vi "Read_Coil_Traces.vi"(1 "Reduction":i32=10, 2 "New Folder":path, 3 "Gas Desk Folder":path) -> ()   [LabVIEW 2010]
uses:
  Controls/Ch_and_Spans.ctl
  Globals/Meas_global.vi
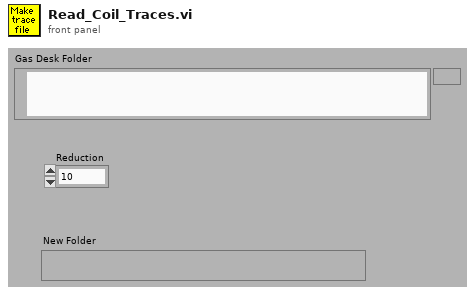
[diagram p1: front panel]
types:
  T1 = typedef "Ch_and_Spans.ctl" = cluster{"high limit (10V)":sgl, "low limit (-10V)":sgl, "Ch No":i16, "Var name":string, "Use Latest Calib":bool}
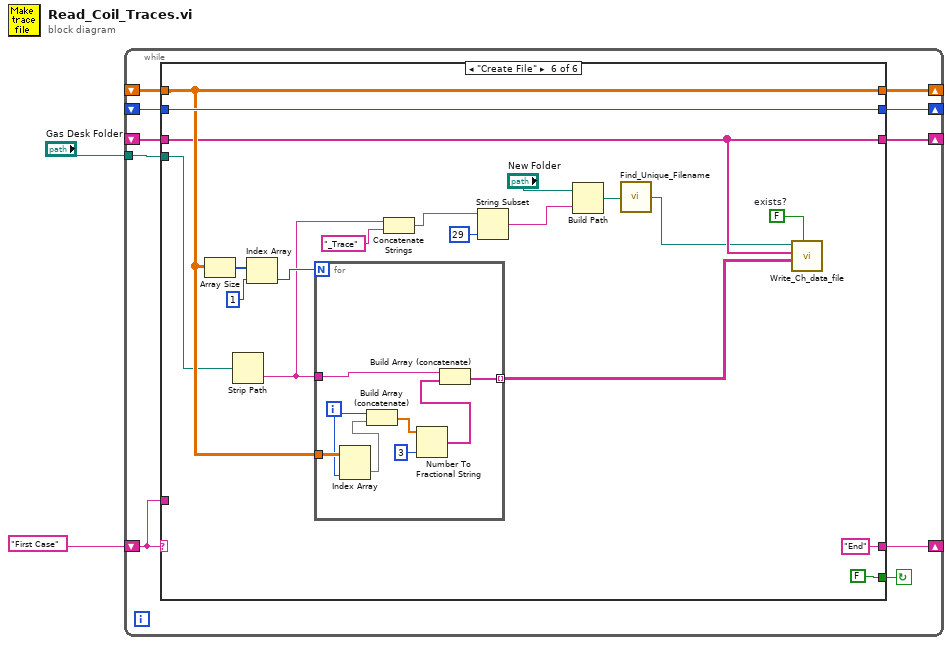
[diagram p0: block diagram]
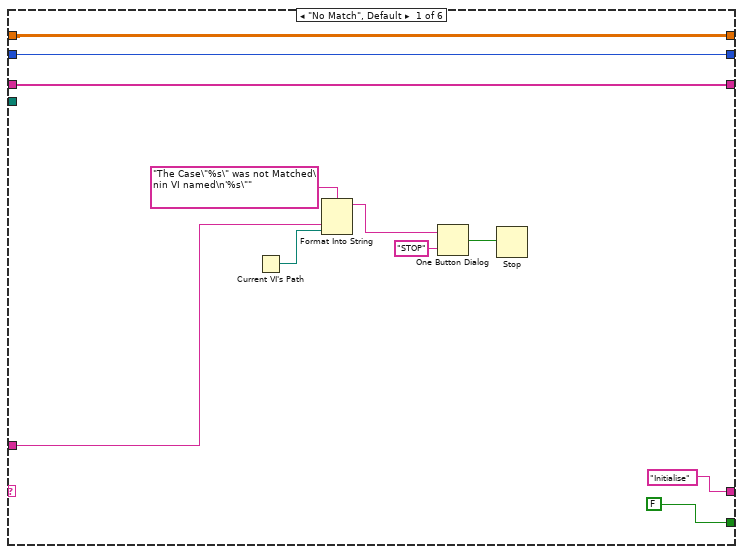
[diagram p2: hidden frame]
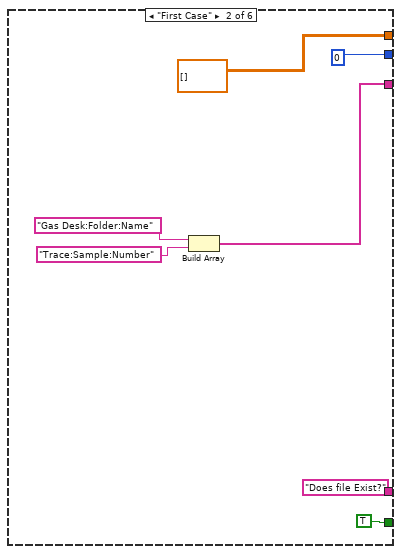
[diagram p3: hidden frame]
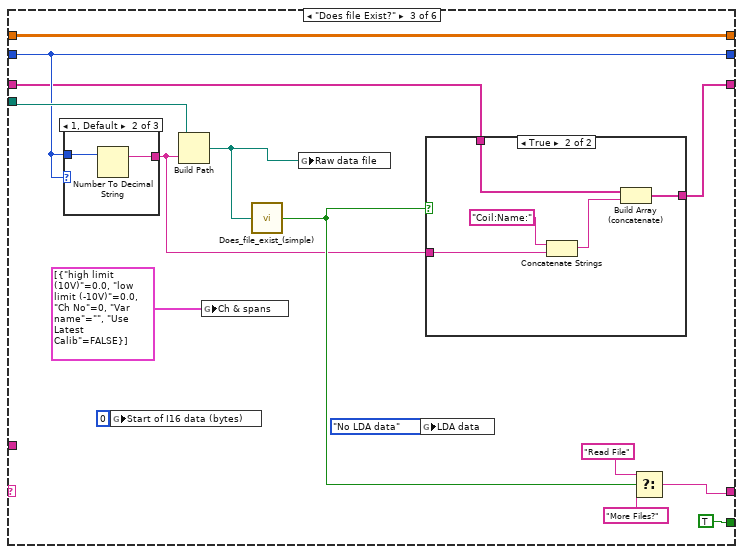
[diagram p4: hidden frame]
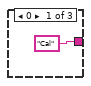
[diagram p6: hidden frame]
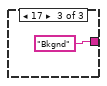
[diagram p7: hidden frame]
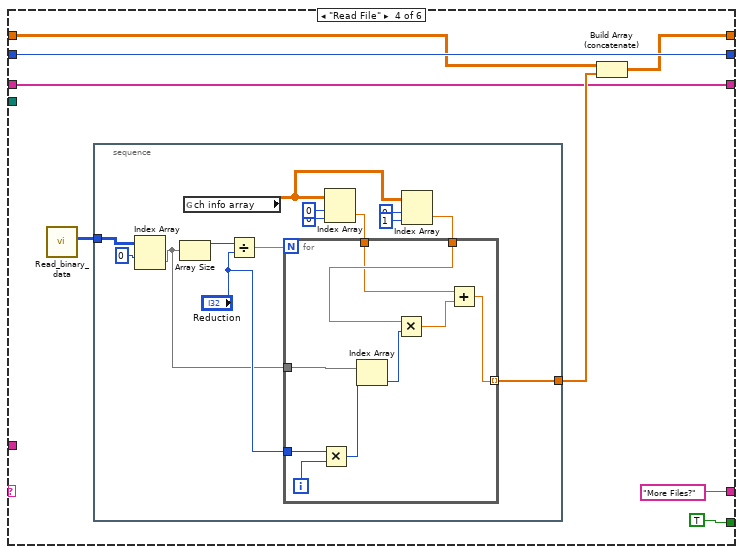
[diagram p8: hidden frame]
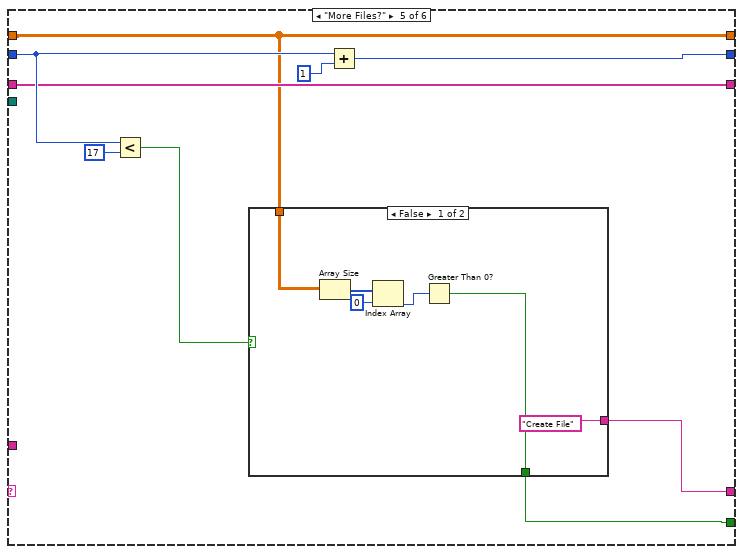
[diagram p9: hidden frame]
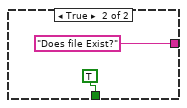
[diagram p10: hidden frame]
diagram:
  n1 = while {
    shift-left: "First Case" -> [w10]
    shift-right: [w11] -> _
    shift-right: [w9] -> _
    shift-left: _ -> [w7]
    tunnel: "Gas Desk Folder" -> [w8]
    shift-right: [w6] -> _
    shift-left: _ -> [w5]
    shift-right: [w3] -> _
    shift-left: _ -> [w4]
    stop <- w12 continue-if-true
    n2 = case shown="\"Create File\"" w10 {
      tunnel: [FALSE TRUE TRUE TRUE w87 FALSE] -> w12
      tunnel: ["Initialise" "Does file Exist?" w41 "More Files?" w90 "End"] -> w11
      tunnel: w10 -> [w18 _ _ _ _ _]
      tunnel: [w14 0 w35 w62 w92 w121] -> w9
      tunnel: w8 -> [_ _ w44 _ _ w116]
      tunnel: w7 -> [w14 _ w35 w62 w94 w121]
      tunnel: [w15 dbl[][] [] w39 w58 w88 w117] -> w6
      tunnel: w5 -> [w15 _ w39 w59 w88 w117]
      tunnel: [w13 w24 w31 w56 w89 w114] -> w3
      tunnel: w4 -> [w13 _ w32 w56 w89 w114]
      frame "No Match", Default {
        n3 = Current VI's Path() -> (path=w17:path)
        n4 = Format Into String(format string="The Case\"%s\" was not Matched\nin VI named\n'%s\"" ("Format String"), w18, w17) -> (resulting string=w21:string)  [unwired: 2 in, 1 out]
        n5 = One Button Dialog(message=w21, button name ("OK")="STOP") -> (true=w19:bool)
        n6 = Stop(stop? (T)=w19) -> ()
      }
      frame "First Case" {
        n7 = Build Array("Gas Desk:Folder:Name", "Trace:Sample:Number") -> (w24:string[])
      }
      frame "Does file Exist?" {
        n8 = case shown="1, Default" w35 {
          tunnel: ["Cal" w54 "Bkgnd"] -> w33
          tunnel: w35 -> [_ w53 _]
          frame 0 {
          }
          frame 1, Default {
            n9 = Number To Decimal String(number=w53) -> (decimal integer string=w54:string)  [unwired: 1 out]
          }
          frame 17 {
          }
        }
        n10 = global write "Meas_global.vi" "Start of I16 data (bytes)"(0 ("Start of I16 data (bytes)")) -> ()
        n11 = Build Path(base path=w44, name or relative path=w33) -> (appended path=w40:path)
        n12 = global write "Meas_global.vi" "Ch & spans"(T1[] [{"high limit (10V)"=0.0, "low limit (-10V)"=0.0, "Ch No"=0, "Var name"="", "Use Latest Calib"=FALSE}] ("Ch & spans")) -> ()
        n13 = call "Does_file_exist_(simple).vi"("Pathname"=w40) -> ("exists?"=w34:bool)
        n14 = global write "Meas_global.vi" "Raw data file"(w40) -> ()
        n15 = global write "Meas_global.vi" "LDA data"(enum16{"No LDA data", "Take LDA data"}."No LDA data" ("LDA data")) -> ()
        n16 = case shown="True" w34 {
          tunnel: w33 -> [_ w50]
          tunnel: w32 -> [w46 w48]
          tunnel: [w46 w47] -> w31
          frame False {
          }
          frame True {
            n17 = Concatenate Strings("Coil:Name:", w50) -> (w49:string)
            n18 = Build Array (concatenate)(w48, w49) -> (w47:string[])
          }
        }
        n19 = Select(t="Read File", s=w34, f="More Files?") -> (s? t:f=w41:string)
      }
      frame "Read File" {
        n20 = call "Read_binary_data.vi"() -> ("Analogue Binary"=w61:i16[][])  [unwired: 9 out]
        n21 = stacked-sequence {
          tunnel: w61 -> [w77]
          tunnel: [w71] -> w60
          frame #0 {
            n22 = Index Array(array=w77, index (row)=0) -> (element=w72:i16[])  [unwired: 1 in]
            n23 = Array Size(array=w72) -> (size(s)=w75:i32)
            n24 = global read "Meas_global.vi" "ch info array"() -> (w66:dbl[][])
            n25 = Divide(x=w75, y="Reduction") -> (x/y=w74:dbl)
            n26 = Index Array(array=w66, index (row)=0, index (col)=0 ("disabled index (col)")) -> (element=w64:dbl)
            n27 = Index Array(array=w66, index (row)=0, index (col)=1 ("disabled index (col)")) -> (element=w65:dbl)
            n28 = for {
              N: w74 -> [_]
              tunnel: "Reduction" -> [w85]
              tunnel: w72 -> [w84]
              tunnel: [w78] -> w71 mode=indexing
              tunnel: w65 -> [w80]
              tunnel: w64 -> [w79]
              i -> [w86]
              n29 = Multiply(x=w85, y=w86) -> (x*y=w83:i32)
              n30 = Index Array(array=w84, index=w83) -> (element=w81:i16)
              n31 = Multiply(x=w80, y=w81) -> (x*y=w82:dbl)
              n32 = Add(x=w79, y=w82) -> (x+y=w78:dbl)
            }
          }
        }
        n33 = Build Array (concatenate)(w59, w60) -> (w58:dbl[][])
      }
      frame "More Files?" {
        n34 = Less?(x=w94, y=17) -> (x < y?=w91:bool)
        n35 = case shown="False" w91 {
          tunnel: ["Create File" "Does file Exist?"] -> w90
          tunnel: w88 -> [w101 _]
          tunnel: [w97 TRUE] -> w87
          frame False {
            n36 = Array Size(array=w101) -> (size(s)=w100:i32[])
            n37 = Index Array(array=w100, index=0) -> (element=w98:i32)
            n38 = Greater Than 0?(x=w98) -> (x > 0?=w97:bool)
          }
          frame True {
          }
        }
        n39 = Add(x=w94, y=1) -> (x+y=w92:i32)
      }
      frame "Create File" {
        w112 = FALSE  # exists?
        n40 = Array Size(array=w117) -> (size(s)=w120:i32[])
        n41 = Strip Path(path=w116) -> (name=w110:string)  [unwired: 1 out]
        n42 = Index Array(array=w120, index=1) -> (element=w118:i32)
        n43 = for {
          N: w118 -> [_]
          tunnel: w117 -> [w130]
          tunnel: w110 -> [w129]
          tunnel: [w124] -> w115 mode=indexing
          i -> [w128]
          n44 = Index Array(array=w130, index (col)=w128) -> (element=w127:dbl[])  [unwired: 1 in]
          n45 = Build Array (concatenate)(w128, w127) -> (w126:dbl[])
          n46 = Number To Fractional String(number=w126, precision (6)=i16 3) -> (F-format string=w125:string[])  [unwired: 2 out]
          n47 = Build Array (concatenate)(w129, w125) -> (w124:string[])
        }
        n48 = Concatenate Strings(w110, "_Trace" ("string")) -> (w108:string)
        n49 = String Subset(string=w108, length (rest)=29 ("length (rest)")) -> (substring=w106:string)  [unwired: 1 out]
        n50 = Build Path(base path="New Folder", name or relative path=w106) -> (appended path=w105:path)
        n51 = call "Find_Unique_Filename.vi"("Path In"=w105) -> ("Unique Path Out"=w104:path)  [unwired: 1 in, 1 out]
        n52 = call "Write_Ch_data_file.vi"("exists?"=w112, "Channel Values"=w115, "Channel names"=w114, "Filename"=w104) -> ()  [unwired: 4 in, 4 out]
      }
    }
  }
